vi "Query Software Licence And Option.vi"(0 "VISA resource name":refnum<visa-resource-name>, 5 "License Type (0:Software Information)":u16(ring) items=["Software License", "Software and Option Information"], 11 "error in (no error)":errorcluster) -> (4 "VISA resource name out":refnum<visa-resource-name>, 6 "Total Number Of Licensed Software":i32, 8 "Licensed Software Information":T1(array[cluster]), 10 "License Option Software Information":T2(array[cluster]), 15 "error out":errorcluster)   [LabVIEW 2020, in "Anritsu Signal Analyzer Series.lvlib"]
doc: "Queries licensed software information including options."
uses:
  Anritsu Signal Analyzer Series.lvlib
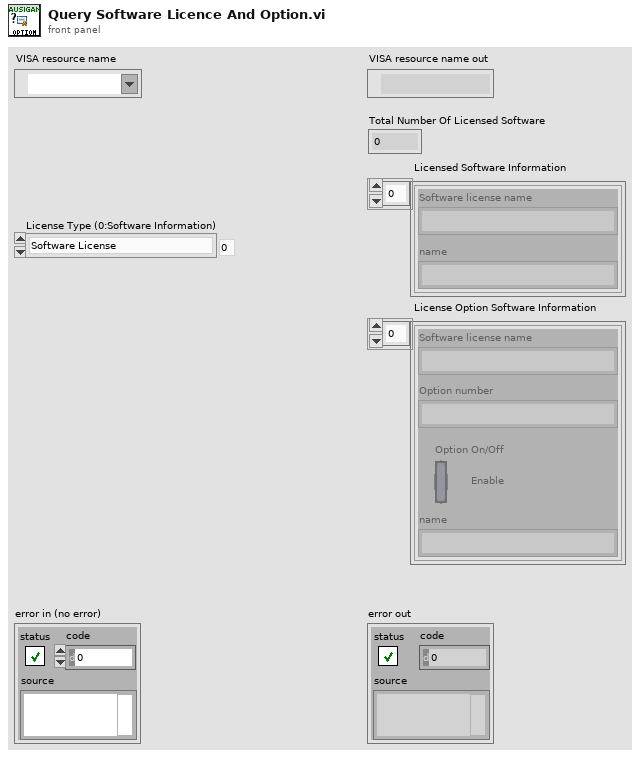
[diagram p1: front panel]
types:
  T1 = cluster{"Software license name":string, "name":string}[]
  T2 = cluster{"Software license name":string, "Option number":string, "Option On/Off":bool, "name":string}[]
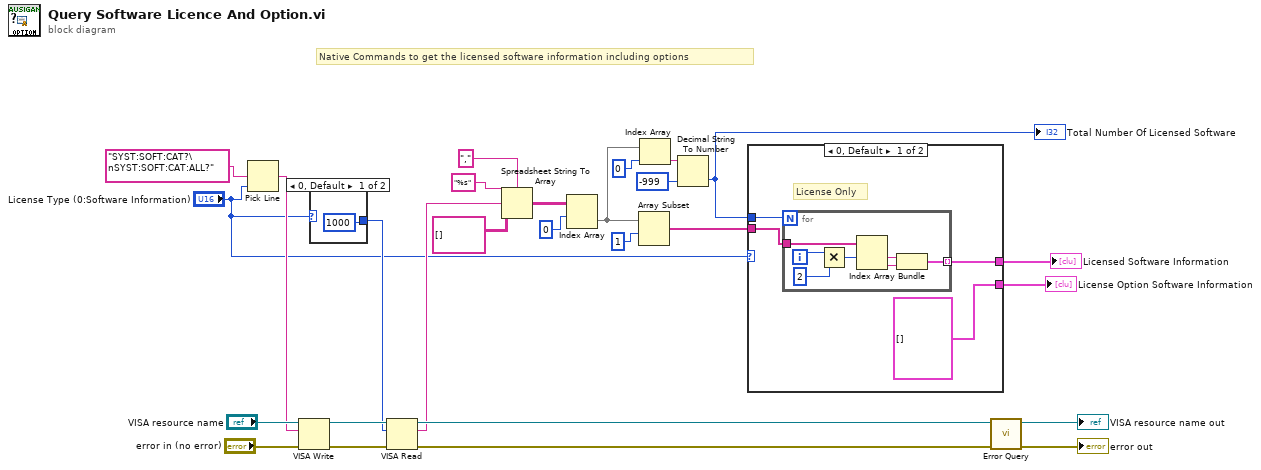
[diagram p0: block diagram]
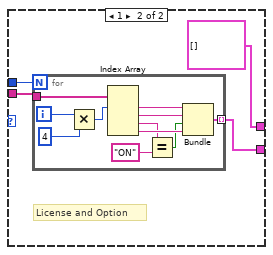
[diagram p2: hidden frame]
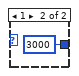
[diagram p3: hidden frame]
diagram:
  # "Native Commands to get the licensed software information including options"
  n1 = Pick Line(multi-line string="SYST:SOFT:CAT?\nSYST:SOFT:CAT:ALL?", line index="License Type (0:Software Information)") -> (output string=w4:string)  [unwired: 1 in]
  n2 = VISA Write(VISA resource name="VISA resource name", write buffer=w4, error in (no error)="error in (no error)") -> (VISA resource name out=w25:refnum<visa-resource-name>, error out=w24:errorcluster)  [unwired: 1 out]
  n3 = case shown="0, Default" "License Type (0:Software Information)" {
    tunnel: [u32 1000 ("byte count (0)") u32 3000 ("byte count (0)")] -> w3
    frame 0, Default {
    }
    frame 1 {
    }
  }
  n4 = VISA Read(VISA resource name=w25, byte count=w3, error in (no error)=w24) -> (VISA resource name out=w20:refnum<visa-resource-name>, read buffer=w19:string, error out=w21:errorcluster)  [unwired: 1 out]
  n5 = Spreadsheet String To Array(delimiter (Tab)=",", format string="%s", spreadsheet string=w19, array type (2D Dbl)=string[][] []) -> (array=w15:string[][])
  n6 = Index Array(array=w15, index (row)=0) -> (element=w9:string[])  [unwired: 1 in]
  n7 = Array Subset(array=w9, index=1) -> (w7:string[])  [unwired: 1 in]
  n8 = Index Array(array=w9, index=0) -> (element=w12:string)
  n9 = Decimal String To Number(string=w12, default (0L)=-999 ("default (0 I32)")) -> (number=w10:i32)  [unwired: 1 in, 1 out]
  "Total Number Of Licensed Software" <- w10
  n10 = case shown="0, Default" "License Type (0:Software Information)" {
    tunnel: w10 -> [w30 w44]
    tunnel: w7 -> [w33 w43]
    tunnel: [cluster{string, string, bool, string}[] [] w42] -> w6
    tunnel: [w32 cluster{string, string}[] []] -> w1
    frame 0, Default {
      # "License Only"
      n11 = for {
        N: w30 -> [_]
        tunnel: w33 -> [w40]
        tunnel: [w34] -> w32 mode=indexing
        i -> [w39]
        n12 = Multiply(x=w39, y=2) -> (x*y=w37:i32)
        n13 = Index Array(array=w40, index #1=w37) -> (element #1=w35:string, element #2=w36:string)  [unwired: 1 in]
        n14 = Bundle(w35, w36) -> (w34:cluster{string, string})  [unwired: 1 in]
      }
    }
    frame 1 {
      # "License and Option"
      n15 = for {
        N: w44 -> [_]
        tunnel: w43 -> [w55]
        tunnel: [w49] -> w42 mode=indexing
        i -> [w54]
        n16 = Multiply(x=w54, y=4) -> (x*y=w52:i32)
        n17 = Index Array(array=w55, index #1=w52) -> (element #1=w50:string, element #2=w51:string, element #3=w47:string, element #4=w48:string)  [unwired: 3 in]
        n18 = Equal?(x=w47, y="ON") -> (x = y?=w45:bool)
        n19 = Bundle(w50, w51, w45, w48) -> (w49:cluster{string, string, bool, string})  [unwired: 1 in]
      }
    }
  }
  "License Option Software Information" <- w6
  "Licensed Software Information" <- w1
  n20 = call "Error Query.vi"("error in (no error)"=w21, "VISA resource name"=w20) -> ("error out"=→"error out":errorcluster, "VISA resource name out"=→"VISA resource name out":refnum<visa-resource-name>)  [unwired: 6 in, 2 out]
